vi "add_data.vi"(0 "1-D Array of Real 2":dbl[](array[numeric]), 1 "1-D Array of Real":dbl[](array[numeric]), 2 "Real":dbl) -> ()   [LabVIEW 2012]
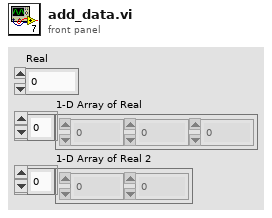
[diagram p1: front panel]
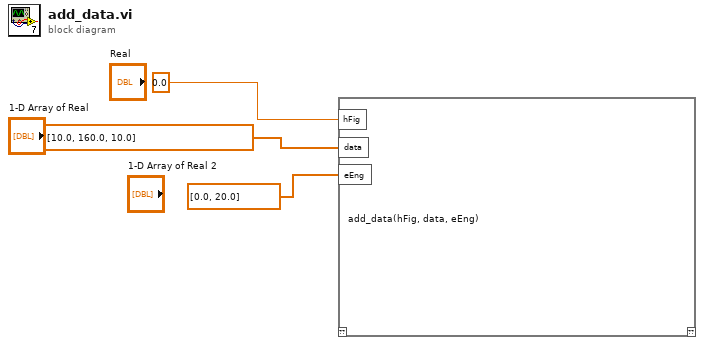
[diagram p0: block diagram]
diagram:
  n1 = script code="add_data(hFig, data, eEng)"("hFig"=0.0 ("Real"), "data"=dbl[] [10.0, 160.0, 10.0] ("1-D Array of Real"), "eEng"=dbl[] [0.0, 20.0] ("1-D Array of Real")) -> ()  [unwired: 1 in, 1 out]
